vi "ZCAN_FilterSheet.vi"(0 "error in (no error)":errorcluster caption="错误输入（无错误）", 2 "can_index_handle":u32, 7 "filter_mode":u32, 9 "Start":u32 caption="起始ID" format="%x", 11 "End":u32 caption="结束ID" format="%x") -> (14 "error out":errorcluster caption="错误输出", 16 "can_index_handle（out）":u32)   [LabVIEW 2011, in "zlgcan.lvlib"]
doc: "设置滤波表格"
uses:
  zlgcan.lvlib
  bin/ControlCANFD.dll
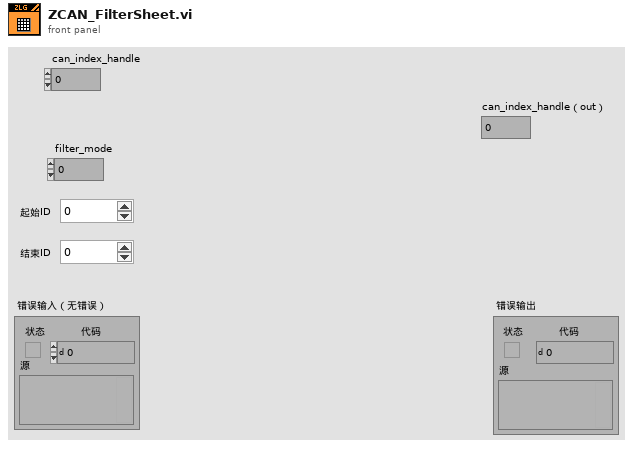
[diagram p1: front panel]
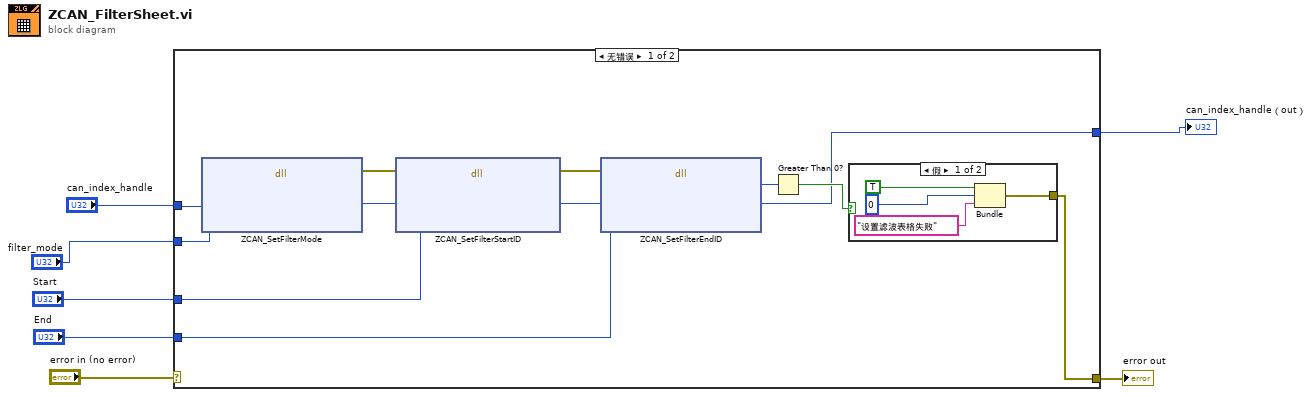
[diagram p0: block diagram]
diagram:
  n1 = case shown="无错误" "error in (no error)" {
    selector: "error in (no error)" -> [_ w24]
    tunnel: [w12 w24] -> w6
    tunnel: "can_index_handle" -> [w15 _]
    tunnel: "filter_mode" -> [w11 _]
    tunnel: "Start" -> [w10 _]
    tunnel: "End" -> [w9 _]
    tunnel: [w8 _] -> w1
    frame No Error {
      n2 = dll-call lib="C:/Users/ttc52/Desktop/DHC FD LV2018/LABIVIEW2011 CANFD Tool_V1.2.4_x86_20250428/bin/ControlCANFD.dll" fn="ZCAN_SetFilterMode"("channel_handle"=w15, "mode"=w11) -> (error out=w16:errorcluster, "channel_handle"=w17:u32)  [unwired: 5 in, 1 out]
      n3 = dll-call lib="C:/Users/ttc52/Desktop/DHC FD LV2018/LABIVIEW2011 CANFD Tool_V1.2.4_x86_20250428/bin/ControlCANFD.dll" fn="ZCAN_SetFilterStartID"(error in=w16, "channel_handle"=w17, "startID"=w10) -> (error out=w19:errorcluster, "channel_handle"=w18:u32)  [unwired: 4 in, 1 out]
      n4 = dll-call lib="C:/Users/ttc52/Desktop/DHC FD LV2018/LABIVIEW2011 CANFD Tool_V1.2.4_x86_20250428/bin/ControlCANFD.dll" fn="ZCAN_SetFilterEndID"(error in=w19, "channel_handle"=w18, "endID"=w9) -> ("return"=w14:u32, "channel_handle"=w8:u32)  [unwired: 3 in, 2 out]
      n5 = Greater Than 0?(x=w14) -> (x > 0?=w13:bool)
      n6 = case shown="假" w13 {
        tunnel: [w20 _] -> w12
        frame False {
          n7 = Bundle("status"=TRUE, "code"=0, "消息"="设置滤波表格失败") -> (w20:cluster{"status":bool, "code":i32, "消息":string})  [unwired: 1 in]
        }
        frame True {
        }
      }
    }
    frame Error {
    }
  }
  "error out" <- w6
  "can_index_handle（out）" <- w1
